vi "_emi_ SMLoop Restart Counter.vi"(0 "Loop Index/Numb":u16, 1 "Action(Get Index)":T1=enum."Get index") -> (4 "Index out":u16, 8 "Numb Restarts":i32, 10 "Size":i32)   [LabVIEW 2011]
uses:
  Loop control/Private/_emi_Loop control int action.ctl
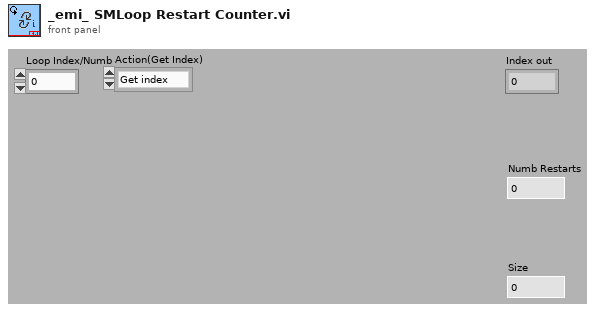
[diagram p1: front panel]
types:
  T1 = typedef "_emi_Loop control int action.ctl" = enum16{"Init index", "Get index", "Set index", "Get Size"}
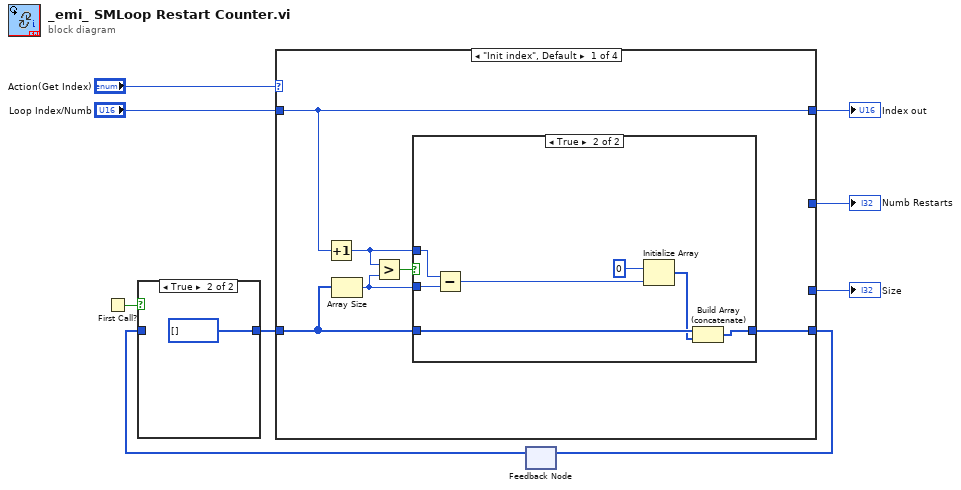
[diagram p0: block diagram]
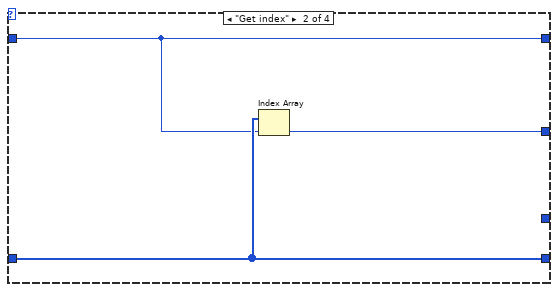
[diagram p3: hidden frame]
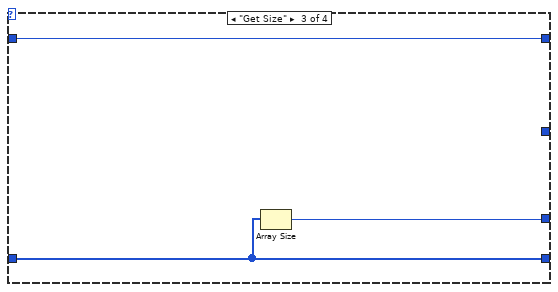
[diagram p4: hidden frame]
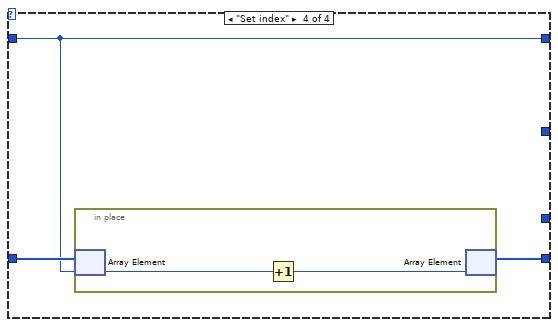
[diagram p5: hidden frame]
diagram:
  n1 = First Call?() -> (First Call?: T/F=w9:bool)
  n2 = feedback #1() -> (w3:i32[])  [unwired: 1 in]
  n3 = case shown="True" w9 {
    tunnel: [w10 i32[] []] -> w4
    tunnel: w3 -> [w10 _]
    frame False {
    }
    frame True {
    }
  }
  n4 = case shown="\"Init index\", Default" "Action(Get Index)" {
    tunnel: [w17 w27 w31 w32] -> w8
    tunnel: "Loop Index/Numb" -> [w17 w27 w31 w32]
    tunnel: [w13 w28 w30 w33] -> w5
    tunnel: w4 -> [w12 w28 w30 w34]
    tunnel: [_ w26 _ _] -> w1
    tunnel: [_ _ w29 _] -> w2
    frame "Init index", Default {
      n5 = Increment(x=w17) -> (x+1=w14:u16)
      n6 = Array Size(array=w12) -> (size(s)=w15:i32)
      n7 = Greater?(x=w14, y=w15) -> (0:w16:bool)
      n8 = case shown="True" w16 {
        tunnel: w15 -> [_ w24]
        tunnel: w14 -> [_ w25]
        tunnel: [w18 w20] -> w13
        tunnel: w12 -> [w18 w22]
        frame False {
        }
        frame True {
          n9 = Subtract(x=w25, y=w24) -> (x-y=w23:i32)
          n10 = Initialize Array(0, w23) -> (w21:i32[])
          n11 = Build Array (concatenate)(w22, w21) -> (w20:i32[])
        }
      }
    }
    frame "Get index" {
      n12 = Index Array(array=w28, index=w27) -> (element=w26:i32)
    }
    frame "Get Size" {
      n13 = Array Size(array=w30) -> (size(s)=w29:i32)
    }
    frame "Set index" {
      n14 = in-place {
        n15 = in-place-array #2(w34, w32) -> (w36:i32)
        n16 = Increment(x=w36) -> (x+1=w35:i32)
        n17 = in-place-array #2(w35) -> (w33:i32[])  [unwired: 1 out]
      }
    }
  }
  "Index out" <- w8
  "Size" <- w2
  "Numb Restarts" <- w1
  n18 = feedback-in #1(w5) -> ()
